vi "pullPatch_v02.vi"(0 "manp in":T2={"Actuator COM"="COM6", "Actuator type"=enum."Scientifica"}, 1 "reset motion":T1=enum."slow_dualPatch", 5 "Current Position":i32[](array[numeric]), 7 "retract distance (um)":dbl=100.0, 9 "retract step size (um)":dbl=5.0, 11 "error in":errorcluster) -> (4 "manip out":T2={"Actuator COM"="COM14", "Actuator type"=enum."Scientifica"}, 15 "error out":errorcluster)   [LabVIEW 2019]
uses:
  pipette cleaning/pressure box/cleaning_soft/controls/actuator_cluster.ctl
  pipette cleaning/pressure box/cleaning_soft/controls/actuator_type.ctl
  controls/scope_motion.ctl
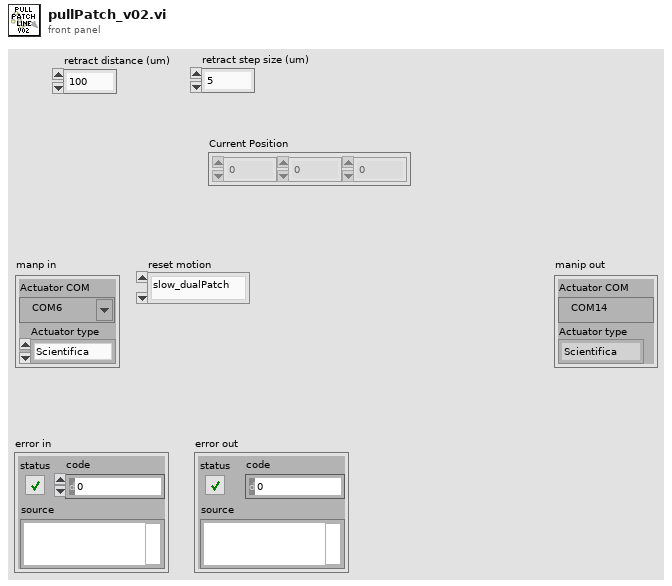
[diagram p1: front panel]
types:
  T1 = typedef "scope_motion.ctl" = enum16{"superSlow", "fast", "slow", "find slice speed", "slow_dualPatch"}
  T2 = typedef "actuator_cluster.ctl" = cluster{"Actuator COM":refnum<visa-resource-name>, "Actuator type":T3}
  T3 = typedef "actuator_type.ctl" = enum16{"Scientifica", "Sutter", "Demo", "Off"}
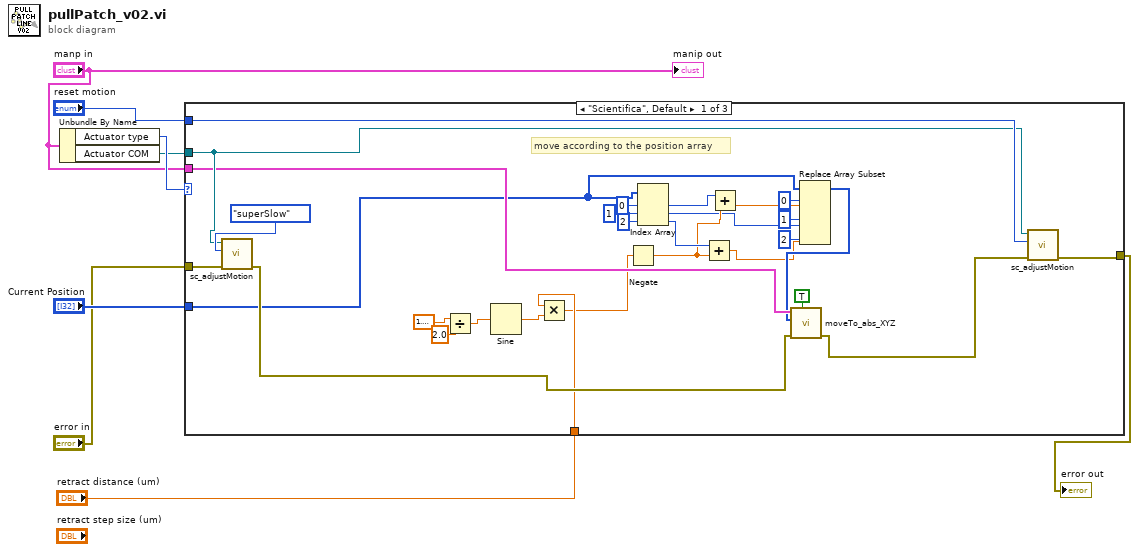
[diagram p0: block diagram]
diagram:
  n1 = Unbundle By Name("manp in") -> ("Actuator type"=w8:T3, "Actuator COM"=w7:refnum<visa-resource-name>)
  n2 = case shown="\"Scientifica\", Default" w8 {
    tunnel: w7 -> [w33 _ _]
    tunnel: "error in" -> [w37 w38 w39]
    tunnel: [w34 w38 w39] -> w5
    tunnel: "reset motion" -> [w36 _ _]
    tunnel: "Current Position" -> [w29 _ _]
    tunnel: "manp in" -> [w32 _ _]
    tunnel: "retract distance (um)" -> [w14 _ _]
    frame "Scientifica", Default {
      # "move according to the position array"
      n3 = call "sc_adjustMotion.vi"("error in (no error)"=w37, "motion"=scope_motion."superSlow", "VISA handle"=w33) -> ("error out"=w31:errorcluster)  [unwired: 7 in, 1 out]
      n4 = Divide(x=1.5707963267948966, y=2.0) -> (x/y=w16:dbl)
      n5 = Sine(x=w16) -> (sin(x)=w18:dbl)
      n6 = Multiply(x=w14, y=w18) -> (x*y=w10:dbl)
      n7 = Negate(x=w10) -> (-x=w11:dbl)
      n8 = Index Array(array=w29, index #1=0 ("index"), index #2=1 ("index"), index #3=2 ("index")) -> (element #1=w12:i32, element #2=w9:i32, element #3=w21:i32)
      n9 = Add(x=w21, y=w11) -> (x+y=w19:dbl)
      n10 = Add(x=w12, y=w11) -> (x+y=w13:dbl)
      n11 = Replace Array Subset(array=w29, new element #1=w13, index #1=0 ("index"), new element #2=w9, index #2=1 ("index"), new element #3=w19, index #3=2 ("index")) -> (w20:i32[])
      n12 = call "moveTo_abs_XYZ.vi"("blocking?"=TRUE, "error in"=w31, "XYZ location (steps)"=w20, "Actuator cluster in"=w32) -> ("error out"=w30:errorcluster)  [unwired: 6 in, 1 out]
      n13 = call "sc_adjustMotion.vi"("error in (no error)"=w30, "motion"=w36, "VISA handle"=w33) -> ("error out"=w34:errorcluster)  [unwired: 7 in, 1 out]
    }
    frame "Sutter" {
    }
    frame "Demo" {
    }
  }
  "error out" <- w5
  "manip out" <- "manp in"
